vi "Get Configuration Settings.vi"(8 "error in (no error)":errorcluster caption="错误输入（无错误）") -> (0 "error out":errorcluster caption="错误输出", 3 "Acquisition and Logging Configuration":T1={"Samples per Read"=100, "Number of Reads to Save"=20, "Number of Channels"=4, "Channel Scale Array"=[1.0, 1.0, 1.0, 1.0], "Channel Names"=[], "Trigger - RMS Value"=0.9999999999999994, "Trigger - Channel"=0, "Trigger - Time (Minute)"=10, "TDMS Properties"=[], "Data File Name"="cRIO_Data", "Date Rate"=20} caption="采集与记录配置" {"Date Rate" items=["51.200 kS/s (NI 9234)"=1, "25.600 kS/s (NI 9234)"=2, "17.067 kS/s (NI 9234)"=3, "12.80 kS/s (NI 9234)"=4, "10.240 kS/s (NI 9234)"=5, "8.533 kS/s (NI 9234)"=6, "7.314 kS/s (NI 9234)"=7, "6.400 kS/s (NI 9234)"=8, "5.689 kS/s (NI 9234)"=9, "5.120 kS/s (NI 9234)"=10, "4.654 kS/s (NI 9234)"=11, "4.267 kS/s (NI 9234)"=12, "3.938 kS/s (NI 9234)"=13, "3.657 kS/s (NI 9234)"=14, "3.413 kS/s (NI 9234)"=15, "3.200 kS/s (NI 9234)"=16, "3.012 kS/s (NI 9234)"=17, "2.845 kS/s (NI 9234)"=18, "2.695 kS/s (NI 9234)"=19, "2.560 kS/s (NI 9234)"=20, "2.438 kS/s (NI 9234)"=21, "2.328 kS/s (NI 9234)"=22, "2.226 kS/s (NI 9234)"=23, "2.133 kS/s (NI 9234)"=24, "2.048 kS/s (NI 9234)"=25, "1.969 kS/s (NI 9234)"=26, "1.896 kS/s (NI 9234)"=27, "1.829 kS/s (NI 9234)"=28, "1.765 kS/s (NI 9234)"=29, "1.707 kS/s (NI 9234)"=30, "1.652 kS/s (NI 9234)"=31]})   [LabVIEW 2013]
uses:
  controls/Acquisition and Logging Configuration.ctl
  controls/TDMS Properties.ctl
  <vilib>/LabVIEW Targets/FPGA/cRIO/shared/nicrio_ModuleControls/nicrio_cRIO-9234_DataRatesRing2.ctl
  <vilib>/Utility/xml.llb/Read From XML File(string).vi
panel:
  # "通道"
  # "保存"
  # "采样"
  # "触发"
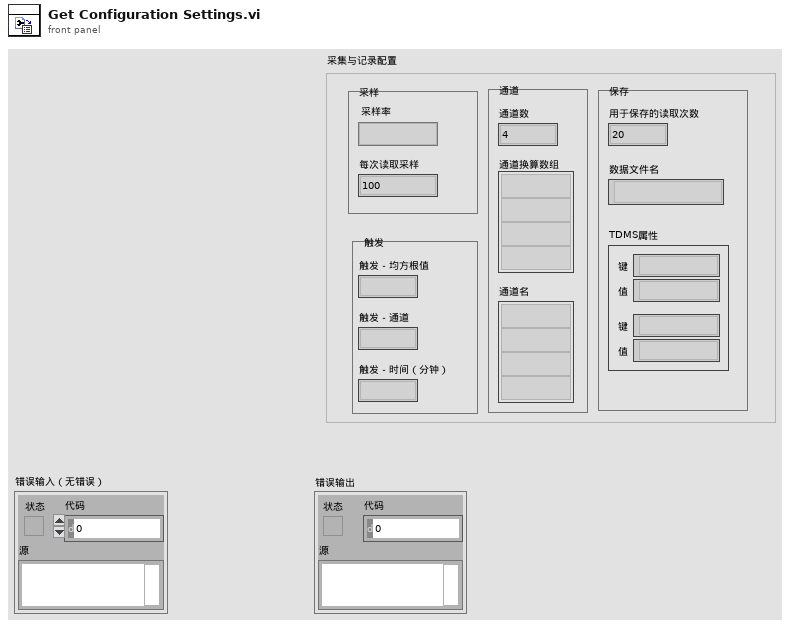
[diagram p1: front panel]
types:
  T1 = typedef "Acquisition and Logging Configuration.ctl" = cluster{"Samples per Read":i32, "Number of Reads to Save":i32, "Number of Channels":i32, "Channel Scale Array":fxp<+,24,12>[], "Channel Names":string[], "Trigger - RMS Value":dbl, "Trigger - Channel":i32, "Trigger - Time (Minute)":i32, "TDMS Properties":T2[], "Data File Name":string, "Date Rate":T3}
  T2 = typedef "TDMS Properties.ctl" = cluster{"Name":string, "Value":string}
  T3 = typedef "nicrio_cRIO-9234_DataRatesRing2.ctl" = u16
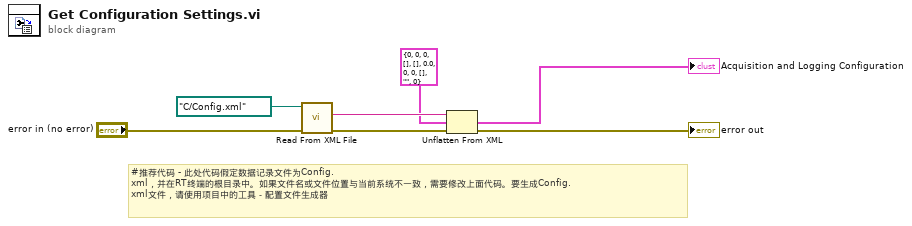
[diagram p0: block diagram]
diagram:
  # "#推荐代码 - 此处代码假定数据记录文件为Config.xml，并在RT终端的根目录中。如果文件名或文件位置与当前系统不一致，需要修改上面代码。要生成Config.xml文件，请使用项目中的工具－配置文件生成器"
  n1 = call-poly <vilib>:"Read From XML File.vi"("error in (no error)"="error in (no error)", "XML File Path"=path "C:/Config.xml") -> ("error out"=w6:errorcluster, "XML Elements"=w5:string)  [unwired: 7 in, 1 out]
  n2 = Unflatten From XML(xml string=w5, type=T1 {"Samples per Read"=0, "Number of Reads to Save"=0, "Number of Channels"=0, "Channel Scale Array"=[], "Channel Names"=[], "Trigger - RMS Value"=0.0, "Trigger - Channel"=0, "Trigger - Time (Minute)"=0, "TDMS Properties"=[], "Data File Name"="", "Date Rate"=0} ("VibLog Configuration"), error in (no error)=w6) -> (value=→"Acquisition and Logging Configuration":T1, error out=→"error out":errorcluster)
